vi "Primary Master.vi"() -> ()   [LabVIEW 2021]
doc: "Primary Modbus master that updates a holding register on the slave at regular intervals as it executes. This provides a secondary master a way to determine to take control of the application should the primary fail."
uses:
  API/Wrapper/Create TCP Master.vi
  Stop Global.vi
  API/Master/Modbus Master.lvclass
  API/Wrapper/API Main.lvlib
panel:
  in  "Operating Mode":u16(ring) items=["Normal", "Simulate Crash"]
  out "Input Register Data":u16[](array[numeric])
  in  "Input Registers to Read":u16[](array[numeric])=[30001, 30002]
  out "Active?":bool
  in  "Heartbeat Register":u16=40001
  in  "Loop Period (ms)":u32=500
  in  "Slave Address":string="localhost"
  # "Primary Modbus Master\n\nReads data from the slave and writes it to shared variables. Periodically writes an incrementing value to a holding register on the slave under normal operation."
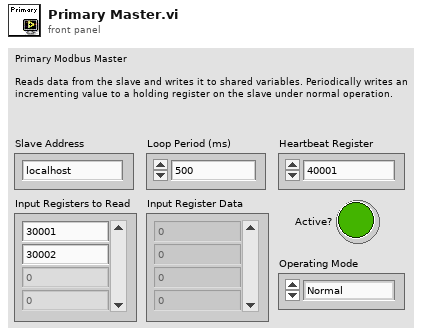
[diagram p1: front panel]
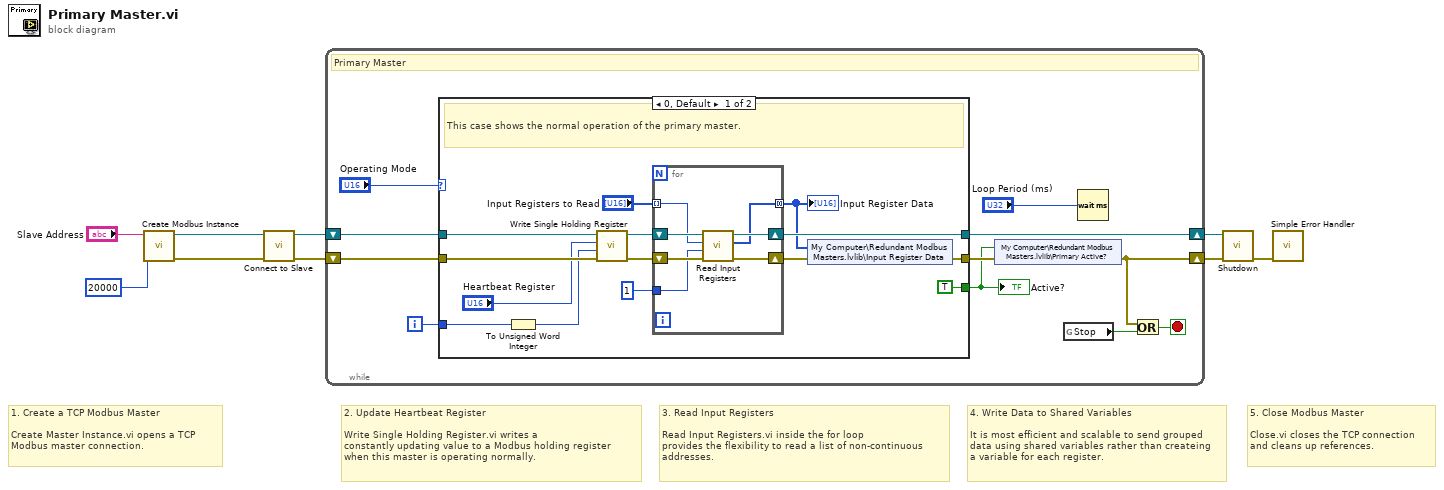
[diagram p0: block diagram]
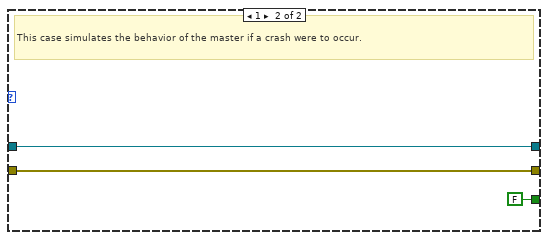
[diagram p2: hidden frame]
diagram:
  # "5. Close Modbus Master\n\nClose.vi closes the TCP connection\nand cleans up references."
  # "4. Write Data to Shared Variables\n\nIt is most efficient and scalable to send grouped\ndata using shared variables rather than createing\na variable for each register."
  # "3. Read Input Registers\n\nRead Input Registers.vi inside the for loop\nprovides the flexibility to read a list of non-continuous\naddresses."
  # "2. Update Heartbeat Register\n\nWrite Single Holding Register.vi writes a \nconstantly updating value to a Modbus holding register \nwhen this master is operating normally."
  # "1. Create a TCP Modbus Master\n\nCreate Master Instance.vi opens a TCP\nModbus master connection."
  n1 = call-poly "Create Modbus Instance.vi"("connect timeout ms"=20000, "address"="Slave Address") -> ("error out"=w1:errorcluster, "TCP master instance"=w2:refnum<class "Modbus Master.lvclass">)  [unwired: 8 in]
  n2 = call-dynamic "Connect to Slave.vi"("error in (no error)"=w1, "Modbus master in"=w2) -> ("error out"=w4:errorcluster, "Modbus master out"=w5:refnum<class "Modbus Master.lvclass">)  [unwired: 8 in]
  n3 = while {
    shift-right: [w17] -> w8
    shift-left: w5 -> [w10]
    shift-right: [w14] -> w7
    shift-left: w4 -> [w20]
    i -> [w19]
    stop <- w16 stop-if-true
    # "Primary Master"
    n4 = case shown="0, Default" "Operating Mode" {
      tunnel: w10 -> [w34 w44]
      tunnel: w20 -> [w33 w43]
      tunnel: w19 -> [w31 _]
      tunnel: [w25 w44] -> w17
      tunnel: [w24 w43] -> w15
      tunnel: [TRUE FALSE] -> w13
      frame 0, Default {
        # "This case shows the normal operation of the primary master."
        n5 = To Unsigned Word Integer(number=w31) -> (unsigned 16bit integer=w30:u16)
        n6 = call-dynamic "Write Single Holding Register.vi"("error in (no error)"=w33, "holding register value"=w30, "address"="Heartbeat Register", "Modbus master in"=w34) -> ("error out"=w28:errorcluster, "Modbus master out"=w29:refnum<class "Modbus Master.lvclass">)  [unwired: 6 in]
        n7 = for {
          shift-right: [w37] -> w25
          shift-left: w29 -> [w41]
          shift-right: [w36] -> w26
          shift-left: w28 -> [w40]
          tunnel: "Input Registers to Read" -> [w39] mode=indexing
          tunnel: u16 1 -> [w38]
          tunnel: [w35] -> w21 mode=concatenating
          n8 = call-dynamic "Read Input Registers.vi"("error in (no error)"=w40, "number of input registers"=w38, "starting address"=w39, "Modbus master in"=w41) -> ("error out"=w36:errorcluster, "register values"=w35:u16[], "Modbus master out"=w37:refnum<class "Modbus Master.lvclass">)  [unwired: 5 in]
        }
        "Input Register Data" <- w21
        n9 = shared-variable "My Computer\\Redundant Modbus Masters.lvlib\\Input Register Data"(w21, error in=w26) -> (error out=w24:errorcluster)
      }
      frame 1 {
        # "This case simulates the behavior of the master if a crash were to occur."
      }
    }
    "Active?" <- w13
    n10 = shared-variable "My Computer\\Redundant Modbus Masters.lvlib\\Primary Active?"(w13, error in=w15) -> (error out=w14:errorcluster)
    n11 = global read "Stop Global.vi" "Stop"() -> (w12:bool)
    n12 = Wait (ms)(milliseconds to wait="Loop Period (ms)") -> ()  [unwired: 1 out]
    n13 = Or(x=w14, y=w12) -> (x .or. y?=w16:bool)
  }
  n14 = call-dynamic "Shutdown.vi"("error in (no error)"=w7, "Modbus master in"=w8) -> ("error out"=w6:errorcluster)  [unwired: 9 in]
  n15 = call <vilib>:"Simple Error Handler.vi"("error in (no error)"=w6) -> ()  [unwired: 4 in, 5 out]
